vi "Read Actor Index.vi"(7 "Actor in":refnum<class "Actor.lvclass">) -> (2 "Actor Index":i32=-1)   [LabVIEW 2020, in "jettl.lvlib" / "Actor Specific.lvlib"]
uses:
  Actor Specific.lvlib
  Actor/Actor.lvclass
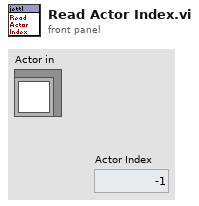
[diagram p1: front panel]
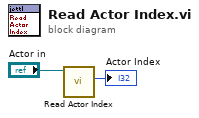
[diagram p0: block diagram]
diagram:
  n1 = call-dynamic "Read Actor Index.vi"("Actor in"="Actor in") -> ("Actor Index"=→"Actor Index":i32)  [unwired: 10 in]
